vi "Problem 15.vi"(11 "Grid Size":u16) -> (3 "Answer":u64)   [LabVIEW 2013, in "Problem 15.lvlib"]
uses:
  Problem 15.lvlib
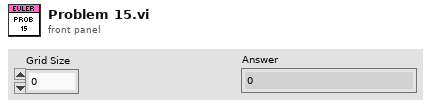
[diagram p1: front panel]
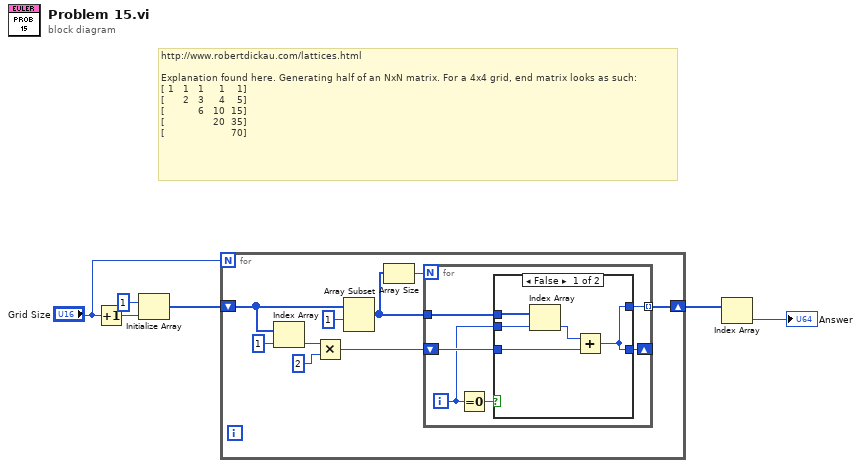
[diagram p0: block diagram]
diagram:
  # "http://www.robertdickau.com/lattices.html\n\nExplanation found here. Generating half of an NxN matrix. For a 4x4 grid, end matrix looks as such:\n[ 1   1   1     1    1]\n[      2   3     4    5]\n[           6   10  15]\n[                20  35]\n[                      70]"
  n1 = Increment(x="Grid Size") -> (x+1=w6:u16)
  n2 = Initialize Array(u64 1 ("element"), w6) -> (w4:u64[])
  n3 = for {
    N: "Grid Size" -> [_]
    shift-right: [w9] -> w2
    shift-left: w4 -> [w12]
    n4 = Index Array(array=w12, index=1) -> (element=w14:u64)
    n5 = Multiply(x=w14, y=u64 2) -> (x*y=w10:u64)
    n6 = Array Subset(array=w12, index=1) -> (w8:u64[])  [unwired: 1 in]
    n7 = Array Size(array=w8) -> (size(s)=w7:i32)
    n8 = for {
      N: w7 -> [_]
      tunnel: w8 -> [w20]
      tunnel: [w18] -> w9 mode=indexing
      shift-right: [w16] -> _
      shift-left: w10 -> [w19]
      i -> [w17]
      n9 = Equal To 0?(x=w17) -> (x = 0?=w21:bool)
      n10 = case shown="False" w21 {
        tunnel: w20 -> [w26 _]
        tunnel: w19 -> [w23 w27]
        tunnel: [w22 w27] -> w18
        tunnel: w17 -> [w25 _]
        tunnel: [w22 w27] -> w16
        frame False {
          n11 = Index Array(array=w26, index=w25) -> (element=w24:u64)
          n12 = Add(x=w24, y=w23) -> (x+y=w22:u64)
        }
        frame True {
        }
      }
    }
  }
  n13 = Index Array(array=w2) -> (element=→"Answer":u64)  [unwired: 1 in]
